vi "Example Test 3.vi"() -> ()   [LabVIEW 2014]
uses:
  <vilib>/measure/NI_MABase.lvlib
panel:
  out "error out 2":errorcluster
  out "myString":string
  out "signal out 2":waveform(dbl)
  in  "b 2":dbl=4.0
  in  "a 2":dbl=3.0
  out "signal out":waveform(dbl)
  out "error out":errorcluster
  in  "error in (no error)":errorcluster
  in  "b":dbl=2.0
  in  "a":dbl=1.0
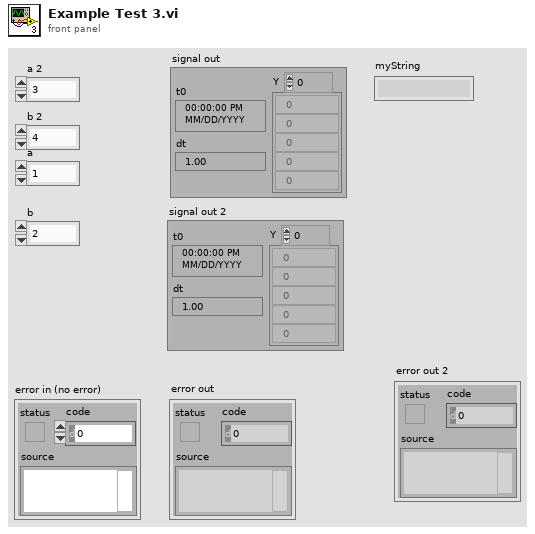
[diagram p1: front panel]
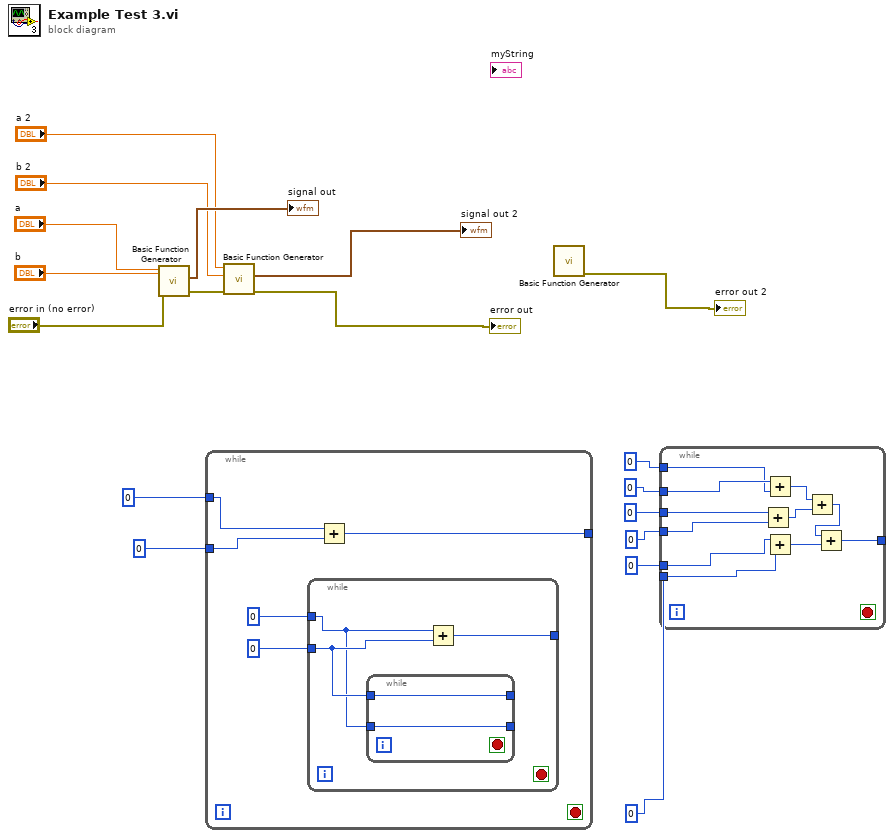
[diagram p0: block diagram]
diagram:
  n1 = call <vilib>:"Basic Function Generator.vi"("error in (no error)"="error in (no error)", "amplitude"="b", "frequency"="a") -> ("error out"=w14:errorcluster, "signal out"=→"signal out":waveform(dbl))  [unwired: 6 in, 1 out]
  n2 = while {
    tunnel: 0 -> [w23]
    tunnel: 0 ("y") -> [w22]
    tunnel: [w21] -> _
    stop <- _ stop-if-true
    n3 = while {
      tunnel: 0 -> [w24]
      tunnel: 0 ("y") -> [w25]
      tunnel: [w26] -> _
      stop <- _ stop-if-true
      n4 = while {
        tunnel: w25 -> [w28]
        tunnel: w24 -> [w27]
        tunnel: [w28] -> _
        tunnel: [w27] -> _
        stop <- _ stop-if-true
      }
      n5 = Add(x=w24, y=w25) -> (x+y=w26:i32)
    }
    n6 = Add(x=w23, y=w22) -> (x+y=w21:i32)
  }
  n7 = call <vilib>:"Basic Function Generator.vi"("error in (no error)"=w14, "amplitude"="b 2", "frequency"="a 2") -> ("error out"=→"error out":errorcluster, "signal out"=→"signal out 2":waveform(dbl))  [unwired: 6 in, 1 out]
  n8 = call <vilib>:"Basic Function Generator.vi"() -> ("error out"=→"error out 2":errorcluster)  [unwired: 9 in, 2 out]
  n9 = while {
    tunnel: 0 -> [w29]
    tunnel: 0 -> [w39]
    tunnel: 0 ("y") -> [w38]
    tunnel: 0 -> [w37]
    tunnel: 0 -> [w36]
    tunnel: 0 ("y") -> [w35]
    tunnel: [w30] -> _
    stop <- _ stop-if-true
    n10 = Add(x=w38, y=w37) -> (x+y=w34:i32)
    n11 = Add(x=w39, y=w29) -> (x+y=w33:i32)
    n12 = Add(x=w36, y=w35) -> (x+y=w32:i32)
    n13 = Add(x=w33, y=w34) -> (x+y=w31:i32)
    n14 = Add(x=w31, y=w32) -> (x+y=w30:i32)
  }
